vi "Send Authorization Request.vi"(8 "error in (no error)":errorcluster, 11 "Connection in":refnum<class "Connection.lvclass">) -> (0 "error out":errorcluster, 1 "timeout":bool, 2 "Authorization":T1, 3 "Connection out":refnum<class "Connection.lvclass">)   [LabVIEW 2013, in "Connection_GOSPL.lvlib" / "Connection.lvclass"]
uses:
  Connection.lvclass
  auth -- cluster.ctl
  Connection.lvclass/Connection.ctl
  <vilib>/LabVIEW Open Source Project/Unicity/RandomStringGenerator/RandomStringGenerator.lvclass
  Store/Store.lvclass
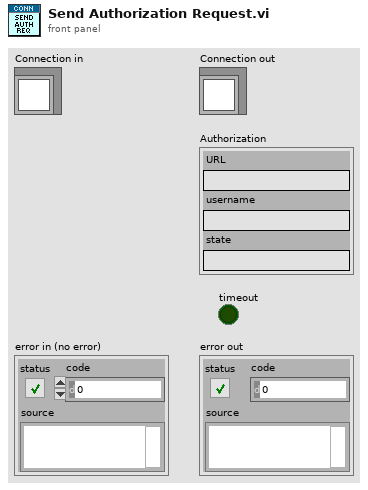
[diagram p1: front panel]
types:
  T1 = typedef "Connection_GOSPL.lvlib/Connection.lvclass/auth -- cluster.ctl" = cluster{"URL":string, "username":string, "state":string}
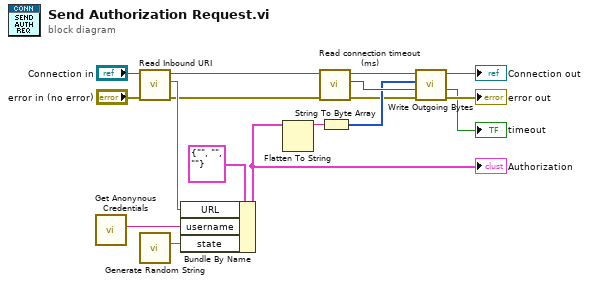
[diagram p0: block diagram]
diagram:
  n1 = call "Get Anonynous Credentials.vi"() -> ("Anonymous username"=w11:string)  [unwired: 10 in, 1 out]
  n2 = call "Read Inbound URI.vi"("Connection in"="Connection in") -> ("Inbound URI"=w12:string, "Connection out"=w3:refnum<class "Connection.lvclass">)  [unwired: 9 in]
  n3 = call <vilib>:"Generate Random String.vi"() -> ("Random String"=w9:string)  [unwired: 11 in]
  n4 = Bundle By Name(cluster=T1 {"URL"="", "username"="", "state"=""} ("Authorization"), "URL"=w12, "username"=w11, "state"=w9) -> (w13:T1)
  "Authorization" <- w13
  n5 = Flatten To String(anything=w13) -> (data string=w6:string)  [unwired: 3 in, 2 out]
  n6 = call "Read connection timeout (ms).vi"("error in (no error)"="error in (no error)", "Connection in"=w3) -> ("error out"=w4:errorcluster, "connection timeout (ms)"=w8:i32, "Connection out"=w2:refnum<class "Connection.lvclass">)  [unwired: 7 in]
  n7 = String To Byte Array(string=w6) -> (unsigned byte array=w7:u8[])
  n8 = call-dynamic "Write Outgoing Bytes.vi"("error in (no error)"=w4, "timeout (2000 ms)"=w8, "Bytes"=w7, "Connection in"=w2) -> ("error out"=→"error out":errorcluster, "timeout"=→"timeout":bool, "Connection out"=→"Connection out":refnum<class "Connection.lvclass">)  [unwired: 5 in]
